vi "TPNT_ReadLogFields.vi"(9 "default":string="name= value", 10 "TPNT_TP":T1={"name"="", "type"="", "algor"=[], "update_rate"=0.0, "Limits"={"Alarm Type"="", "Lower "=0.0, "Upper"=0.0, "Nominal"=0.0, "outrange"=FALSE, "Check"=TRUE, "latch"=FALSE, "level"=""}, "Samples"={"samples"=0, "counter"=0, "Values"=[], "Current Value"="", "filter"="", "precision"=2}, "next_update"=0, "Status"="", "monitor"=TRUE, "error"=FALSE, "Log"={"log"=FALSE, "file"=path "", "type"="", "format"="", "updaterate"=0.0, "nex_update"=0, "mode"=""}, "permissions"="", "ID"=""} {"Log"."updaterate" format="%.2f"; "Samples"."Values" format="%.2f"; "Samples"."samples" min=1 step=1; "Limits"."Nominal" format="%.2f"; "Limits"."Upper" format="%.2f"; "Limits"."Lower" format="%.2f"; "update_rate" format="%.2f"}) -> (2 "message to log":string)   [LabVIEW 2016]
uses:
  TPNT_TP.ctl
  TPNT_Limits.ctl
  TPNT_Samples.ctl
  TPNT_Log.ctl
panel:
  in  "fields":string[](array[string])=["name", "value", "status", "samples"]
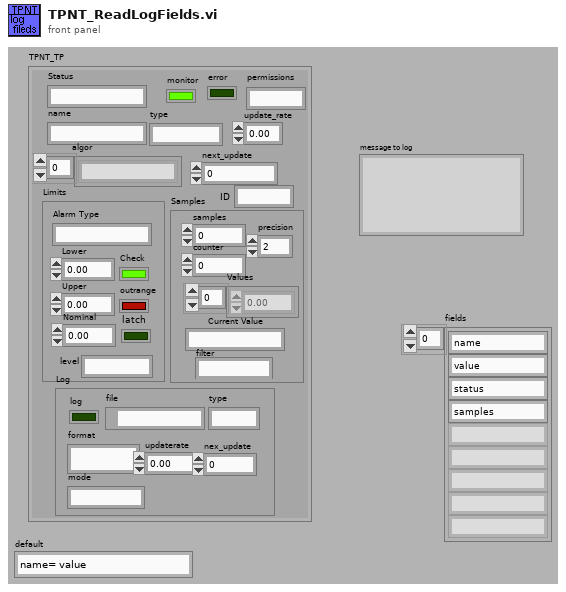
[diagram p1: front panel]
types:
  T1 = typedef "TPNT_TP.ctl" = cluster{"name":string, "type":string, "algor":string[], "update_rate":sgl, "Limits":T2, "Samples":T3, "next_update":u32, "Status":string, "monitor":bool, "error":bool, "Log":T4, "permissions":string, "ID":string}
  T2 = typedef "TPNT_Limits.ctl" = cluster{"Alarm Type":string, "Lower ":dbl, "Upper":dbl, "Nominal":dbl, "outrange":bool, "Check":bool, "latch":bool, "level":string}
  T3 = typedef "TPNT_Samples.ctl" = cluster{"samples":i32, "counter":i32, "Values":dbl[], "Current Value":string, "filter":string, "precision":u8}
  T4 = typedef "TPNT_Log.ctl" = cluster{"log":bool, "file":path, "type":string, "format":string, "updaterate":dbl, "nex_update":u32, "mode":string}
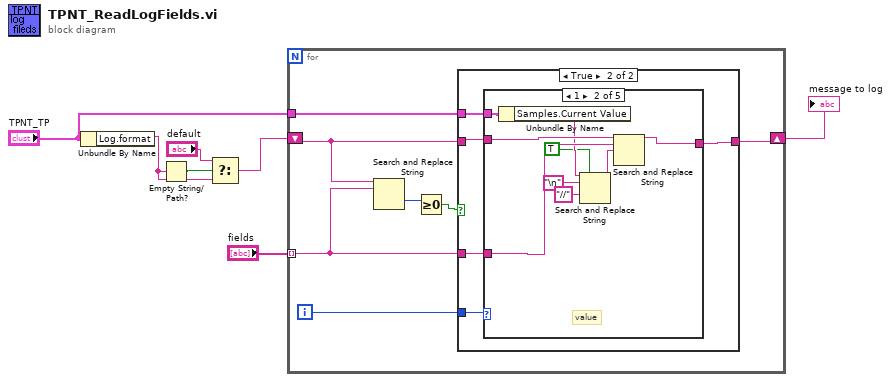
[diagram p0: block diagram]
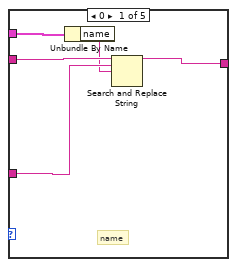
[diagram p3: hidden frame]
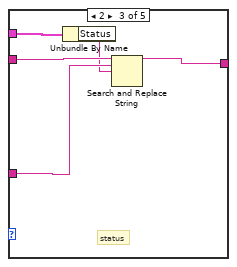
[diagram p4: hidden frame]
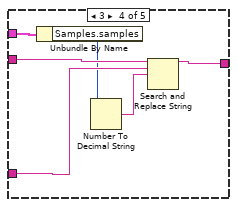
[diagram p5: hidden frame]
diagram:
  n1 = Unbundle By Name("TPNT_TP") -> ("Log.format"=w2:string)
  n2 = Empty String/Path?(string/path=w2) -> (empty?=w4:bool)
  n3 = Select(t="default", s=w4, f=w2) -> (s? t:f=w1:string)
  n4 = for {
    tunnel: "TPNT_TP" -> [w9]
    shift-right: [w10] -> w5
    shift-left: w1 -> [w11]
    tunnel: "fields" -> [w12] mode=indexing
    i -> [w8]
    n5 = Search and Replace String(input string=w11, search string=w12) -> (offset past replacement=w14:i32)  [unwired: 1 in, 8 out]
    n6 = Greater Or Equal To 0?(x=w14) -> (x >= 0?=w13:bool)
    n7 = case shown="True" w13 {
      tunnel: w12 -> [_ w17]
      tunnel: w11 -> [w15 w18]
      tunnel: [w15 w16] -> w10
      tunnel: w9 -> [_ w19]
      tunnel: w8 -> [_ w20]
      frame False {
      }
      frame True {
        n8 = case shown="1" w20 {
          tunnel: w19 -> [w23 w32 w37 w43 _]
          tunnel: w18 -> [w25 w34 w39 w45 w46]
          tunnel: w17 -> [w24 w33 w38 w44 _]
          tunnel: [w21 w31 w35 w42 w46] -> w16
          frame 0 {
            # "name"
            n9 = Unbundle By Name(w23) -> ("name"=w22:string)
            n10 = Search and Replace String(input string=w25, search string=w24, replace string=w22) -> (result string=w21:string)  [unwired: 1 in, 7 out]
          }
          frame 1 {
            # "value"
            n11 = Unbundle By Name(w32) -> ("Samples.Current Value"=w30:string)
            n12 = Search and Replace String(replace all?=TRUE ("replace all? (F)"), input string=w30, search string="\n", replace string="//" ("replace string (\"\")")) -> (result string=w29:string)  [unwired: 1 in, 6 out]
            n13 = Search and Replace String(input string=w34, search string=w33, replace string=w29) -> (result string=w31:string)  [unwired: 1 in, 7 out]
          }
          frame 2 {
            # "status"
            n14 = Unbundle By Name(w37) -> ("Status"=w36:string)
            n15 = Search and Replace String(input string=w39, search string=w38, replace string=w36) -> (result string=w35:string)  [unwired: 1 in, 7 out]
          }
          frame 3 {
            n16 = Unbundle By Name(w43) -> ("Samples.samples"=w41:i32)
            n17 = Number To Decimal String(number=w41) -> (decimal integer string=w40:string)  [unwired: 1 out]
            n18 = Search and Replace String(input string=w45, search string=w44, replace string=w40) -> (result string=w42:string)  [unwired: 1 in, 7 out]
          }
          frame Default {
          }
        }
      }
    }
  }
  "message to log" <- w5
